vi "Find Installs.vi"(8 "error in":errorcluster, 11 "TSDiscovery in":refnum<class "TSDiscovery.lvclass">) -> (0 "error out":errorcluster, 3 "TSInstalls Out":T1[](array[typedef]))   [LabVIEW 2025, in "TSDiscovery.lvclass"]
doc: "Discovers all TestStand installations available on the current system and returns them as an array of TSInstall elements.\n\nThe method is responsible for detecting installed TestStand versions and populating the defined metadata fields (Version, Architecture, Version Key, ID)."
uses:
  TSDiscovery.lvclass
  Type Definitions/TSInstall--cluster.ctl
  Type Definitions/Architecture--enum.ctl
  <vilib>/nisyscfg/Get Installed Components.vi
  <vilib>/nisyscfg/Close (System).vi
  <vilib>/regexp/Match Regular Expression.xnode
  <vilib>/nisyscfg/nisyscfg.lvlib
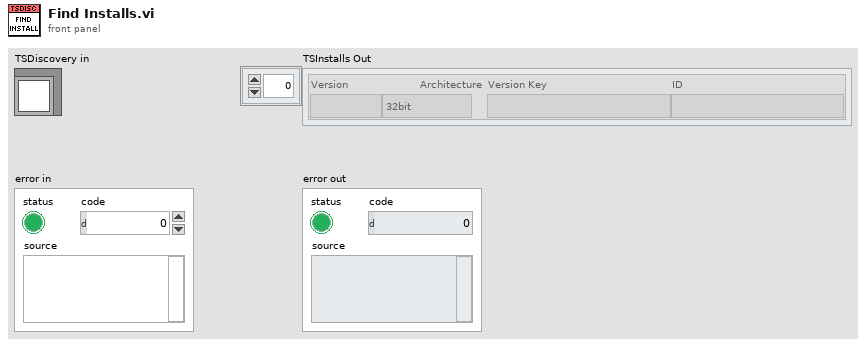
[diagram p1: front panel]
types:
  T1 = typedef "TSInstall--cluster.ctl" = cluster{"Version":string, "Architecture":T2, "Version Key":string, "ID":string}
  T2 = typedef "Architecture--enum.ctl" = enum16{"32bit", "64bit"}
  T3 = typedef "nisyscfg.lvlib/Software 1.2.ctl" = cluster{"title":string, "description":string, "ID":string, "version":string, "component type":T4}
  T4 = typedef "nisyscfg.lvlib/Component Type.ctl" = u32
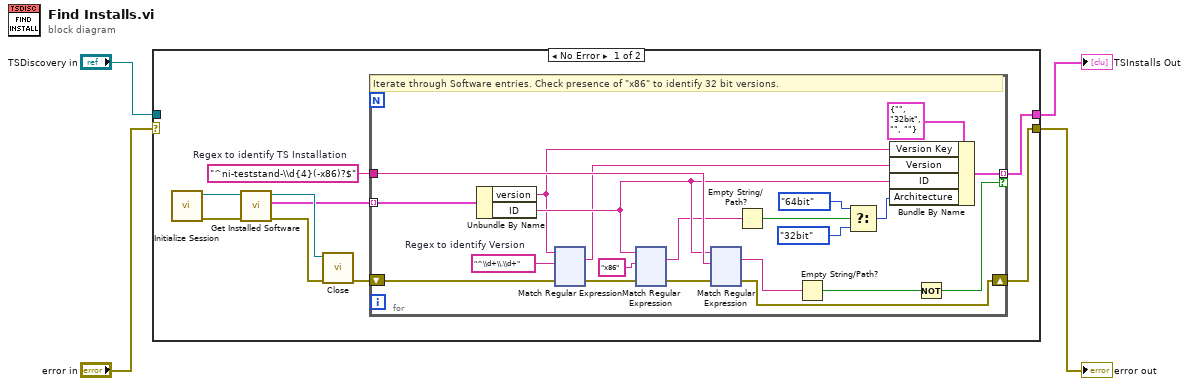
[diagram p0: block diagram]
diagram:
  n1 = case shown="No Error" "error in" {
    selector: "error in" -> [_ w386]
    tunnel: "TSDiscovery in" -> [_ _]
    tunnel: [w5 w386] -> w2
    tunnel: [w6 _] -> w1
    frame No Error {
      w7 = "^ni-teststand-\\d{4}(-x86)?$"  # Regex to identify TS Installation
      n2 = call <vilib>:"Initialize Session.vi"() -> ("error out"=w13:errorcluster, "Session out"=w11:refnum<k21>)  [unwired: 10 in]
      n3 = call-poly <vilib>:"Get Installed Software.vi"("error in (no error)"=w13, "Session in"=w11) -> ("error out"=w12:errorcluster, "Software Components"=w9:T3[], "Session out"=w10:refnum<k21>)  [unwired: 7 in]
      n4 = call-poly <vilib>:"Close.vi"("error in (no error)"=w12, "Session in"=w10) -> ("error out"=w8:errorcluster)  [unwired: 9 in]
      n5 = for {
        tunnel: w9 -> [w34] mode=indexing
        shift-right: [w32] -> w5
        shift-left: w8 -> [w17]
        tunnel: w7 -> [w33]
        tunnel: [w30] -> w6 mode=indexing if=w27
        w18 = "^\\d+\\.\\d+"  # Regex to identify Version
        # "Iterate through Software entries. Check presence of \"x86\" to identify 32 bit versions."
        n6 = Unbundle By Name(w34) -> ("version"=w19:string, "ID"=w26:string)
        n7 = xnode "Match Regular Expression"("input string"=w19, "regular expression"=w18, "error in"=w17) -> ("whole match"=w15:string, "error out"=w16:errorcluster)  [unwired: 3 in, 3 out]
        n8 = xnode "Match Regular Expression"("input string"=w26, "regular expression"="x86", "error in"=w16) -> ("whole match"=w24:string, "error out"=w23:errorcluster)  [unwired: 3 in, 3 out]
        n9 = xnode "Match Regular Expression"("input string"=w26, "regular expression"=w33, "error in"=w23) -> ("whole match"=w29:string, "error out"=w32:errorcluster)  [unwired: 3 in, 3 out]
        n10 = Empty String/Path?(string/path=w24) -> (empty?=w21:bool)
        n11 = Empty String/Path?(string/path=w29) -> (empty?=w28:bool)
        n12 = Select(t=Architecture--enum."64bit" ("Architecture"), s=w21, f=Architecture--enum."32bit" ("Architecture")) -> (s? t:f=w20:T2)
        n13 = Bundle By Name(cluster=T1 {"Version"="", "Architecture"=enum."32bit", "Version Key"="", "ID"=""} ("TSInstall"), "Version Key"=w19, "Version"=w15, "ID"=w26, "Architecture"=w20) -> (w30:T1)
        n14 = Not(x=w28) -> (.not. x?=w27:bool)
      }
    }
    frame Error {
      # "Pass error without further action"
    }
  }
  "TSInstalls Out" <- w1
  "error out" <- w2
